vi "niRFUtil RFHS Benchmark GetData.vi"(0 "BenchTask":T1, 2 "Generate Tree":bool, 11 "error in (no error)":errorcluster) -> (4 "Time":u64[](array[numeric]), 6 "Counters":u64[](array[numeric]), 8 "Frequency":u64, 10 "Tree Names":string[](array[string]), 14 "Tree":string, 15 "error out":errorcluster)   [LabVIEW 2015, in "niRFUtil.lvlib"]
uses:
  niRFUtil.lvlib
  niRFUtil RFHS Benchmark Task.ctl
  niRFUtil RFHS Util Phases.ctl
  kernel32.dll
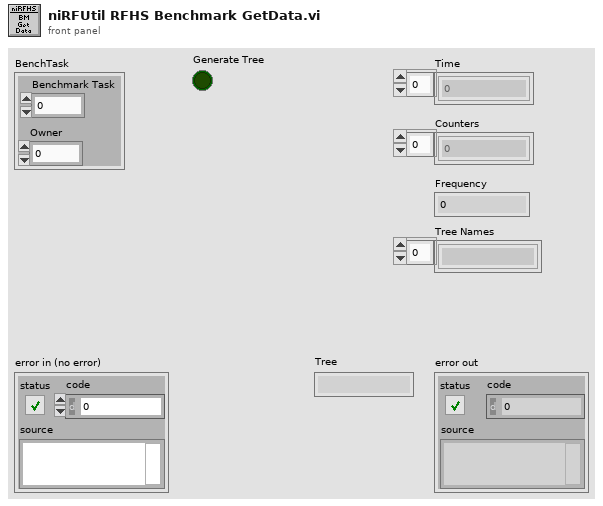
[diagram p1: front panel]
types:
  T1 = typedef "niRFUtil.lvlib/niRFUtil RFHS Benchmark Task.ctl" = cluster{"Benchmark Task":u64, "Owner":u32}
  T2 = typedef "niRFUtil.lvlib/niRFUtil RFHS Util Phases.ctl" = enum32{"Reserved", "CreateBenchmarkTask", "CRC", "UE UL Segment Transport Block", "UE UL Read Buffer", "UE UL TC", "UE UL RM", "UE UL CI", "Scramble", "Group Bits", "Benchmark Task Start", "Benchmark Task Stop", "Descramble", "Deinterleave", "eNB UL HARQ", "eNB UL Read Buffer", "eNB UL AFEM", "eNB UL Turbo Decoder", "Get Benchmark Task Data", "G31", "UL Gen Freq2Time", "Gen Power Spectrum", "UL Ana Time2Freq", "Benchmark Task Enter", "Benchmark Task Leave"}
  T3 = typedef "niRFUtil.lvlib/niRFUtil RFHS Benchmark TaskMgrInfo.ctl" = cluster{"Name":string, "Owner":i32, "ID":i32}
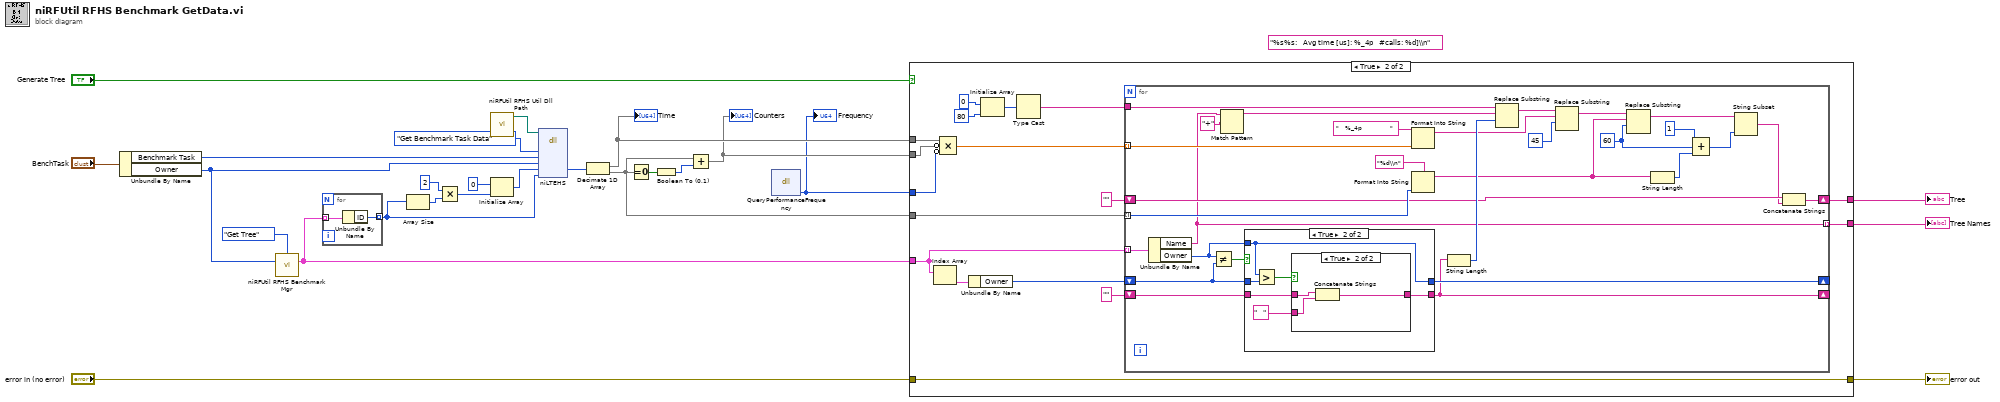
[diagram p0: block diagram]
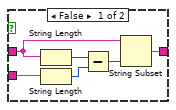
[diagram p4: hidden frame]
diagram:
  (unwired) "%s%s:   Avg time [us]: %_4p   #calls: %d]\\n" ("format string")
  n1 = Unbundle By Name("BenchTask") -> ("Benchmark Task"=w17:u64, "Owner"=w15:u32)
  n2 = call "niRFUtil RFHS Benchmark Mgr.vi"("What"=enum16{"Register", "Get Tree"}."Get Tree", "Owner"=w15) -> ("Tree"=w9:T3[])  [unwired: 12 in, 1 out]
  n3 = for {
    tunnel: w9 -> [w27] mode=indexing
    tunnel: [w26] -> w14 mode=indexing
    n4 = Unbundle By Name(w27) -> ("ID"=w26:i32)
  }
  n5 = Array Size(array=w14) -> (size(s)=w3:i32)
  n6 = Multiply(x=2 ("y"), y=w3) -> (x*y=w16:i32)
  n7 = call "niRFUtil RFHS Util Dll Path.vi"() -> ("Path"=w25:path)  [unwired: 7 in, 4 out]
  n8 = Initialize Array(u64 0 ("element"), w16) -> (w22:u64[])
  n9 = dll-call lib="C:/ni-rt/system/HPCExecBenchDll.dll" fn="niLTEHS"(path in=w25, "what"=niRFUtil_RFHS_Util_Phases."Get Benchmark Task Data" ("Enum"), "benchmarkTask"=w17, "benchId"=w15, "buffer"=w22, "IDs"=w14) -> ("buffer"=w21:u64[])  [unwired: 7 in, 2 out]
  n10 = Decimate 1D Array(w21) -> (w12:u64[], w13:u64[])
  "Time" <- w12
  n11 = Equal To 0?(x=w13) -> (x = 0?=w20:bool[])
  n12 = Boolean To (0,1)(Boolean=w20) -> (0, 1=w19:i16[])
  n13 = Add(x=w13, y=w19) -> (x+y=w11:u64[])
  "Counters" <- w11
  n14 = dll-call lib="kernel32.dll" fn="QueryPerformanceFrequency"() -> ("frequency"=w10:u64)  [unwired: 5 in, 2 out]
  "Frequency" <- w10
  n15 = case shown="True" "Generate Tree" {
    tunnel: w13 -> [_ w45]
    tunnel: w12 -> [_ w40]
    tunnel: w11 -> [_ w39]
    tunnel: w10 -> [_ w38]
    tunnel: w9 -> [_ w36]
    tunnel: [_ w35] -> w7
    tunnel: [_ w34] -> w6
    tunnel: "error in (no error)" -> [w28 w29]
    tunnel: [w28 w29] -> w1
    frame False {
    }
    frame True {
      n16 = Index Array(array=w36) -> (element=w42:T3)  [unwired: 1 in]
      n17 = Compound Arithmetic op=MULTIPLY(w40, invert w39, invert w38) -> (w37:dbl[])
      n18 = Unbundle By Name(w42) -> ("Owner"=w41:i32)
      n19 = Initialize Array(u8 0 ("element"), 80 ("dimension size")) -> (w31:u8[])
      n20 = Type Cast(x=w31) -> (*(type *) &x=w30:string)  [unwired: 1 in]
      n21 = for {
        tunnel: w36 -> [w69] mode=indexing
        tunnel: w45 -> [w59] mode=indexing
        shift-right: [w67] -> _
        shift-left: "" -> [w70]
        shift-right: [w49] -> w35
        shift-left: "" -> [w51]
        shift-right: [w71] -> _
        shift-left: w41 -> [w72]
        tunnel: w37 -> [w62] mode=indexing
        tunnel: [w48] -> w34 mode=indexing
        tunnel: w30 -> [w68]
        w54 = 60 ("offset (0)")
        n22 = Unbundle By Name(w69) -> ("Name"=w48:string, "Owner"=w73:i32)
        n23 = Not Equal?(x=w73, y=w72) -> (x != y?=w74:bool)
        n24 = Match Pattern(string=w48, regular expression="+") -> (before substring=w47:string)  [unwired: 1 in, 3 out]
        n25 = case shown="True" w74 {
          tunnel: [w75 w82] -> w67
          tunnel: w70 -> [w75 w81]
          tunnel: w73 -> [_ w77]
          tunnel: w72 -> [w76 w80]
          tunnel: [w76 w77] -> w71
          frame False {
          }
          frame True {
            n26 = Greater?(x=w77, y=w80) -> (0:w79:bool)
            n27 = case shown="True" w79 {
              tunnel: [w86 w91] -> w82
              tunnel: w81 -> [w88 w90]
              tunnel: "   " -> [w87 w89]
              frame False {
                n28 = String Length(string=w88) -> (length=w83:i32)
                n29 = String Length(string=w87) -> (length=w84:i32)
                n30 = Subtract(x=w83, y=w84) -> (x-y=w85:i32)
                n31 = String Subset(string=w88, length (rest)=w85) -> (substring=w86:string)  [unwired: 1 in]
              }
              frame True {
                n32 = Concatenate Strings(w90, w89) -> (w91:string)
              }
            }
          }
        }
        n33 = Format Into String(format string="   %_4p              ", w62) -> (resulting string=w64:string)  [unwired: 2 in, 1 out]
        n34 = Format Into String(format string="%d\\n", w59) -> (resulting string=w56:string)  [unwired: 2 in, 1 out]
        n35 = String Length(string=w67) -> (length=w66:i32)
        n36 = Replace Substring(3:w66, 4:w47, 5:w68) -> (1:w65:string)  [unwired: 1 in, 1 out]
        n37 = Replace Substring(3:45 ("offset (0)"), 4:w64, 5:w65) -> (1:w58:string)  [unwired: 1 in, 1 out]
        n38 = Replace Substring(3:w54, 4:w56, 5:w58) -> (1:w57:string)  [unwired: 1 in, 1 out]
        n39 = String Length(string=w56) -> (length=w55:i32)
        n40 = Compound Arithmetic op=ADD(1 ("value"), w54, w55) -> (w52:i32)
        n41 = String Subset(string=w57, length (rest)=w52) -> (substring=w50:string)  [unwired: 1 in]
        n42 = Concatenate Strings(w51, w50) -> (w49:string)
      }
    }
  }
  "error out" <- w1
  "Tree" <- w7
  "Tree Names" <- w6
